vi "Autonomous Independent Vision.vi"   [LabVIEW 2016]
doc: "This VI is called when autonomous begins, and will automatically be terminated when autonomous ends. You can carry out timed or sensor driven robot movement independently without needing to return to the caller."
uses:
  Robot Global Data.vi
panel:
  # "Be sure to right-click and choose Data Operations>>Make Current Value default if you want to save the array values with the VI"
types:
  T1 = cluster{"Position":cluster{"x":sgl, "y":sgl}, "Angle":sgl, "Scale":sgl, "Score":sgl, "Bounding Box":cluster{"x":sgl, "y":sgl}[]}[]
  T2 = cluster{"Position":cluster{"x":sgl, "y":sgl}, "Angle":sgl, "Scale":sgl, "Score":sgl, "Bounding Box":cluster{"x":sgl, "y":sgl}[]}
  T3 = typedef "WPI_MotorControlDeviceRef.ctl" = cluster{"DeviceStatus":errorcluster, "Type":T4, "PWM":cluster{"PWM Channel":T5, "DeadBand":T6}, "CAN":cluster{"Device Number":u8, "SetOutput VI Ref":variant, "GetOutput VI Ref":variant, "Enable VI Ref":variant, "Disable VI Ref":variant, "Data":variant}, "Invert":bool}
  T4 = typedef "WPI_MotorControlType.ctl" = enum16{"PWM", "CAN"}
  T5 = typedef "FPGA_DIOPWMChannel.ctl" = enum8{"PWM 0", "PWM 1", "PWM 2", "PWM 3", "PWM 4", "PWM 5", "PWM 6", "PWM 7", "PWM 8", "PWM 9", "PWM MXP 0", "PWM MXP 1", "PWM MXP 2", "PWM MXP 3", "PWM MXP 4", "PWM MXP 5", "PWM MXP 6", "PWM MXP 7", "PWM MXP 8", "PWM MXP 9", "Invalid"}
  T6 = typedef "WPI_PWMDeadband.ctl" = cluster{"Name":string, "maxPositivePwm":i32, "minPositivePwm":i32, "centerPwm":i32, "maxNegativePwm":i32, "minNegativePwm":i32, "angularRange":u16}
  T7 = typedef "WPI_EncoderDevRef.ctl" = cluster{"DevStatus":errorcluster, "EncoderIndex":T8, "CounterIndex":T9, "DistancePerCount":dbl, "Decoding Type":T10}
  T8 = typedef "FPGA_EncoderIdx.ctl" = enum8{"Enc 0", "Enc 1", "Enc 2", "Enc 3", "Enc 4", "Enc 5", "Enc 6", "Enc 7", "Invalid"}
  T9 = typedef "FPGA_CounterCtrSystemIndex.ctl" = enum8{"Ctr 0", "Ctr 1", "Ctr 2", "Ctr 3", "Ctr 4", "Ctr 5", "Ctr 6", "Ctr 7", "Invalid"}
  T10 = typedef "WPI_EncoderType.ctl" = enum16{"1x", "2x", "4x"}
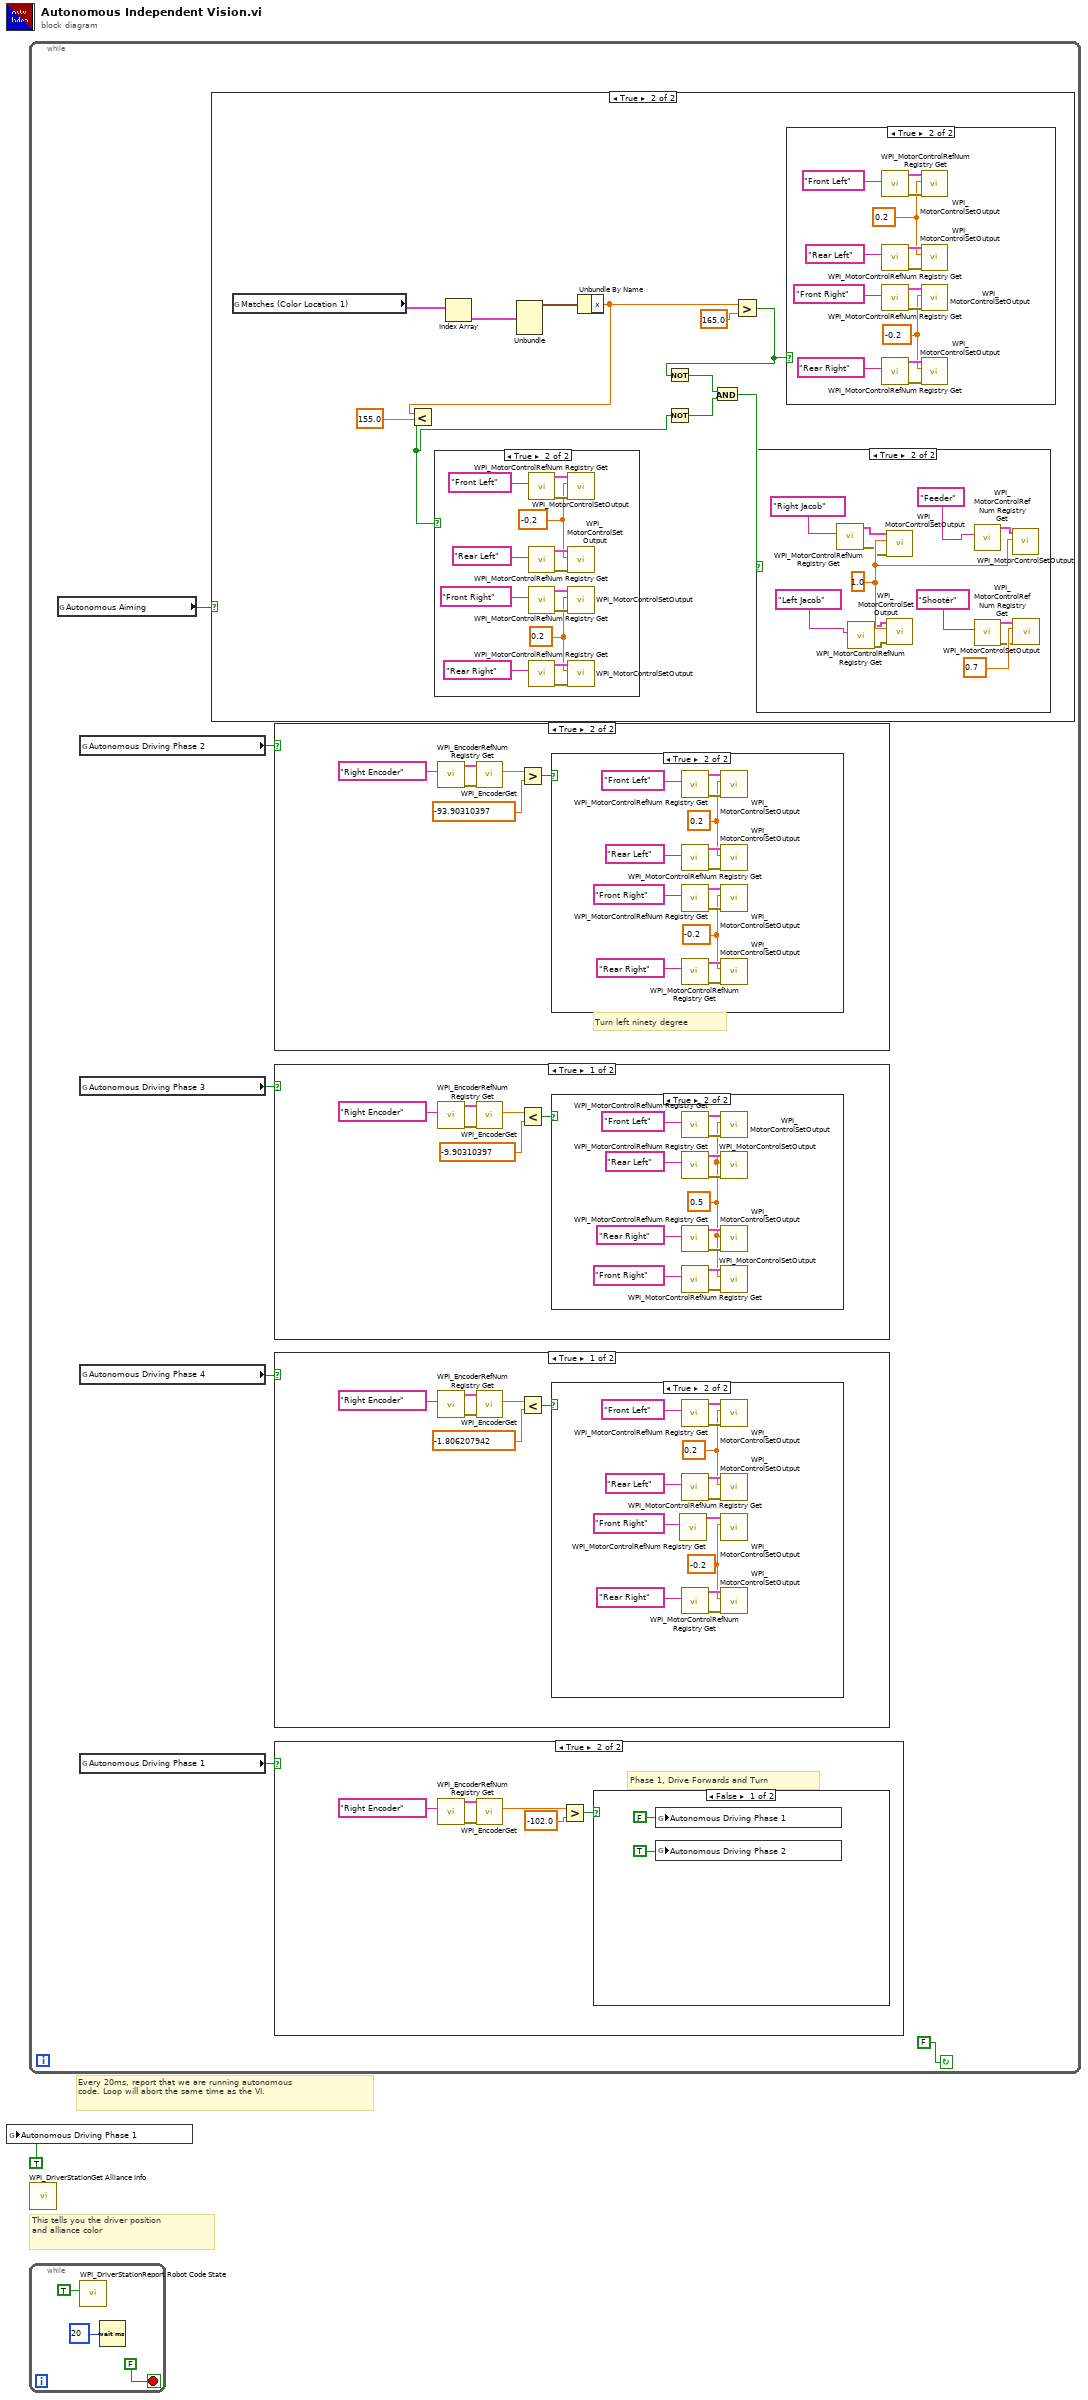
[diagram p0: block diagram]
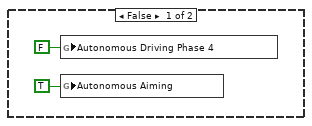
[diagram p2: hidden frame]
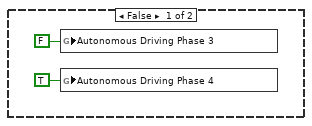
[diagram p4: hidden frame]
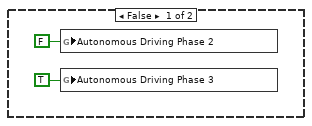
[diagram p7: hidden frame]
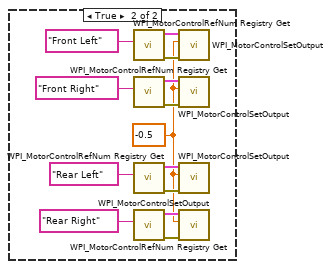
[diagram p13: hidden frame]
diagram:
  # "Every 20ms, report that we are running autonomous\ncode. Loop will abort the same time as the VI."
  # "This tells you the driver position\nand alliance color"
  n1 = global write "Robot Global Data.vi" "Autonomous Driving Phase 1"(TRUE ("Autonomous Driving")) -> ()
  n2 = while {
    stop <- FALSE continue-if-true
    n3 = global read "Robot Global Data.vi" "Autonomous Aiming"() -> (w5:bool)
    n4 = global read "Robot Global Data.vi" "Autonomous Driving Phase 2"() -> (w4:bool)
    n5 = global read "Robot Global Data.vi" "Autonomous Driving Phase 3"() -> (w3:bool)
    n6 = global read "Robot Global Data.vi" "Autonomous Driving Phase 4"() -> (w2:bool)
    n7 = global read "Robot Global Data.vi" "Autonomous Driving Phase 1"() -> (w6:bool)
    n8 = case shown="True" w5 {
      frame False {
      }
      frame True {
        n9 = global read "Robot Global Data.vi" "Matches (Color Location 1)"() -> (w82:T1)
        n10 = Index Array(array=w82) -> (element=w81:T2)  [unwired: 1 in]
        n11 = Unbundle(w81) -> ("Position"=w80:cluster{"x":sgl, "y":sgl})  [unwired: 4 out]
        n12 = Unbundle By Name(w80) -> ("x"=w78:sgl)
        n13 = Less?(x=w78, y=sgl 155.0) -> (x < y?=w75:bool)
        n14 = case shown="True" w75 {
          frame False {
          }
          frame True {
            w99 = 0.2
            w96 = -0.2
            n15 = call <vilib>:"WPI_MotorControlRefNum Registry Get.vi"("refnum name"="Front Left") -> ("error out"=w109:errorcluster, "MotorControlDevRef"=w97:T3)  [unwired: 9 in]
            n16 = call <vilib>:"WPI_MotorControlRefNum Registry Get.vi"("refnum name"="Rear Left") -> ("error out"=w105:errorcluster, "MotorControlDevRef"=w104:T3)  [unwired: 9 in]
            n17 = call <vilib>:"WPI_MotorControlRefNum Registry Get.vi"("refnum name"="Front Right") -> ("error out"=w108:errorcluster, "MotorControlDevRef"=w107:T3)  [unwired: 9 in]
            n18 = call <vilib>:"WPI_MotorControlRefNum Registry Get.vi"("refnum name"="Rear Right") -> ("error out"=w102:errorcluster, "MotorControlDevRef"=w101:T3)  [unwired: 9 in]
            n19 = call <vilib>:"WPI_MotorControlSetOutput.vi"("error in (no error)"=w109, "Output"=w96, "MotorControlDevRef"=w97) -> ()  [unwired: 6 in, 3 out]
            n20 = call <vilib>:"WPI_MotorControlSetOutput.vi"("error in (no error)"=w105, "Output"=w96, "MotorControlDevRef"=w104) -> ()  [unwired: 6 in, 3 out]
            n21 = call <vilib>:"WPI_MotorControlSetOutput.vi"("error in (no error)"=w108, "Output"=w99, "MotorControlDevRef"=w107) -> ()  [unwired: 6 in, 3 out]
            n22 = call <vilib>:"WPI_MotorControlSetOutput.vi"("error in (no error)"=w102, "Output"=w99, "MotorControlDevRef"=w101) -> ()  [unwired: 6 in, 3 out]
          }
        }
        n23 = Not(x=w75) -> (.not. x?=w73:bool)
        n24 = Greater?(x=w78, y=sgl 165.0) -> (0:w76:bool)
        n25 = Not(x=w76) -> (.not. x?=w74:bool)
        n26 = And(x=w74, y=w73) -> (x .and. y?=w72:bool)
        n27 = case shown="True" w72 {
          frame False {
          }
          frame True {
            w95 = 1.0
            n28 = call <vilib>:"WPI_MotorControlRefNum Registry Get.vi"("refnum name"="Right Jacob") -> ("error out"=w93:errorcluster, "MotorControlDevRef"=w92:T3)  [unwired: 9 in]
            n29 = call <vilib>:"WPI_MotorControlRefNum Registry Get.vi"("refnum name"="Left Jacob") -> ("error out"=w88:errorcluster, "MotorControlDevRef"=w87:T3)  [unwired: 9 in]
            n30 = call <vilib>:"WPI_MotorControlSetOutput.vi"("error in (no error)"=w93, "Output"=w95, "MotorControlDevRef"=w92) -> ()  [unwired: 6 in, 3 out]
            n31 = call <vilib>:"WPI_MotorControlSetOutput.vi"("error in (no error)"=w88, "Output"=w95, "MotorControlDevRef"=w87) -> ()  [unwired: 6 in, 3 out]
            n32 = call <vilib>:"WPI_MotorControlRefNum Registry Get.vi"("refnum name"="Feeder") -> ("MotorControlDevRef"=w89:T3)  [unwired: 9 in, 1 out]
            n33 = call <vilib>:"WPI_MotorControlRefNum Registry Get.vi"("refnum name"="Shootér") -> ("error out"=w85:errorcluster, "MotorControlDevRef"=w84:T3)  [unwired: 9 in]
            n34 = call <vilib>:"WPI_MotorControlSetOutput.vi"("Output"=w95, "MotorControlDevRef"=w89) -> ()  [unwired: 7 in, 3 out]
            n35 = call <vilib>:"WPI_MotorControlSetOutput.vi"("error in (no error)"=w85, "Output"=0.7, "MotorControlDevRef"=w84) -> ()  [unwired: 6 in, 3 out]
          }
        }
        n36 = case shown="True" w76 {
          frame False {
          }
          frame True {
            w113 = -0.2
            w110 = 0.2
            n37 = call <vilib>:"WPI_MotorControlRefNum Registry Get.vi"("refnum name"="Front Left") -> ("error out"=w123:errorcluster, "MotorControlDevRef"=w111:T3)  [unwired: 9 in]
            n38 = call <vilib>:"WPI_MotorControlRefNum Registry Get.vi"("refnum name"="Rear Left") -> ("error out"=w119:errorcluster, "MotorControlDevRef"=w118:T3)  [unwired: 9 in]
            n39 = call <vilib>:"WPI_MotorControlRefNum Registry Get.vi"("refnum name"="Front Right") -> ("error out"=w122:errorcluster, "MotorControlDevRef"=w121:T3)  [unwired: 9 in]
            n40 = call <vilib>:"WPI_MotorControlRefNum Registry Get.vi"("refnum name"="Rear Right") -> ("error out"=w116:errorcluster, "MotorControlDevRef"=w115:T3)  [unwired: 9 in]
            n41 = call <vilib>:"WPI_MotorControlSetOutput.vi"("error in (no error)"=w123, "Output"=w110, "MotorControlDevRef"=w111) -> ()  [unwired: 6 in, 3 out]
            n42 = call <vilib>:"WPI_MotorControlSetOutput.vi"("error in (no error)"=w119, "Output"=w110, "MotorControlDevRef"=w118) -> ()  [unwired: 6 in, 3 out]
            n43 = call <vilib>:"WPI_MotorControlSetOutput.vi"("error in (no error)"=w122, "Output"=w113, "MotorControlDevRef"=w121) -> ()  [unwired: 6 in, 3 out]
            n44 = call <vilib>:"WPI_MotorControlSetOutput.vi"("error in (no error)"=w116, "Output"=w113, "MotorControlDevRef"=w115) -> ()  [unwired: 6 in, 3 out]
          }
        }
      }
    }
    n45 = case shown="True" w4 {
      frame False {
      }
      frame True {
        # "Turn left ninety degree"
        n46 = call <vilib>:"WPI_EncoderRefNum Registry Get.vi"("refnum name"="Right Encoder") -> ("error out"=w54:errorcluster, "EncoderDevRef"=w53:T7)  [unwired: 9 in]
        n47 = call <vilib>:"WPI_EncoderGet.vi"("error in (no error)"=w54, "EncoderDevRef"=w53) -> ("Distance"=w52:dbl)  [unwired: 4 in, 5 out]
        n48 = Greater?(x=w52, y=-93.90310397) -> (0:w50:bool)
        n49 = case shown="True" w50 {
          frame False {
            n50 = global write "Robot Global Data.vi" "Autonomous Driving Phase 2"(FALSE ("Autonomous Driving Phase 2")) -> ()
            n51 = global write "Robot Global Data.vi" "Autonomous Driving Phase 3"(TRUE ("Autonomous Driving Phase 3")) -> ()
          }
          frame True {
            w58 = -0.2
            w59 = 0.2
            n52 = call <vilib>:"WPI_MotorControlRefNum Registry Get.vi"("refnum name"="Front Left") -> ("error out"=w71:errorcluster, "MotorControlDevRef"=w70:T3)  [unwired: 9 in]
            n53 = call <vilib>:"WPI_MotorControlRefNum Registry Get.vi"("refnum name"="Rear Left") -> ("error out"=w65:errorcluster, "MotorControlDevRef"=w64:T3)  [unwired: 9 in]
            n54 = call <vilib>:"WPI_MotorControlRefNum Registry Get.vi"("refnum name"="Front Right") -> ("error out"=w68:errorcluster, "MotorControlDevRef"=w67:T3)  [unwired: 9 in]
            n55 = call <vilib>:"WPI_MotorControlRefNum Registry Get.vi"("refnum name"="Rear Right") -> ("error out"=w62:errorcluster, "MotorControlDevRef"=w61:T3)  [unwired: 9 in]
            n56 = call <vilib>:"WPI_MotorControlSetOutput.vi"("error in (no error)"=w71, "Output"=w59, "MotorControlDevRef"=w70) -> ()  [unwired: 6 in, 3 out]
            n57 = call <vilib>:"WPI_MotorControlSetOutput.vi"("error in (no error)"=w65, "Output"=w59, "MotorControlDevRef"=w64) -> ()  [unwired: 6 in, 3 out]
            n58 = call <vilib>:"WPI_MotorControlSetOutput.vi"("error in (no error)"=w68, "Output"=w58, "MotorControlDevRef"=w67) -> ()  [unwired: 6 in, 3 out]
            n59 = call <vilib>:"WPI_MotorControlSetOutput.vi"("error in (no error)"=w62, "Output"=w58, "MotorControlDevRef"=w61) -> ()  [unwired: 6 in, 3 out]
          }
        }
      }
    }
    n60 = case shown="True" w3 {
      frame True {
        n61 = call <vilib>:"WPI_EncoderRefNum Registry Get.vi"("refnum name"="Right Encoder") -> ("error out"=w34:errorcluster, "EncoderDevRef"=w33:T7)  [unwired: 9 in]
        n62 = call <vilib>:"WPI_EncoderGet.vi"("error in (no error)"=w34, "EncoderDevRef"=w33) -> ("Distance"=w31:dbl)  [unwired: 4 in, 5 out]
        n63 = Less?(x=w31, y=-9.90310397) -> (x < y?=w29:bool)
        n64 = case shown="True" w29 {
          frame False {
            n65 = global write "Robot Global Data.vi" "Autonomous Driving Phase 3"(FALSE ("Autonomous Driving Phase 2")) -> ()
            n66 = global write "Robot Global Data.vi" "Autonomous Driving Phase 4"(TRUE ("Autonomous Driving Phase 3")) -> ()
          }
          frame True {
            w37 = 0.5
            n67 = call <vilib>:"WPI_MotorControlRefNum Registry Get.vi"("refnum name"="Front Left") -> ("error out"=w49:errorcluster, "MotorControlDevRef"=w48:T3)  [unwired: 9 in]
            n68 = call <vilib>:"WPI_MotorControlRefNum Registry Get.vi"("refnum name"="Rear Left") -> ("error out"=w43:errorcluster, "MotorControlDevRef"=w42:T3)  [unwired: 9 in]
            n69 = call <vilib>:"WPI_MotorControlRefNum Registry Get.vi"("refnum name"="Rear Right") -> ("error out"=w40:errorcluster, "MotorControlDevRef"=w39:T3)  [unwired: 9 in]
            n70 = call <vilib>:"WPI_MotorControlRefNum Registry Get.vi"("refnum name"="Front Right") -> ("error out"=w46:errorcluster, "MotorControlDevRef"=w45:T3)  [unwired: 9 in]
            n71 = call <vilib>:"WPI_MotorControlSetOutput.vi"("error in (no error)"=w49, "Output"=w37, "MotorControlDevRef"=w48) -> ()  [unwired: 6 in, 3 out]
            n72 = call <vilib>:"WPI_MotorControlSetOutput.vi"("error in (no error)"=w43, "Output"=w37, "MotorControlDevRef"=w42) -> ()  [unwired: 6 in, 3 out]
            n73 = call <vilib>:"WPI_MotorControlSetOutput.vi"("error in (no error)"=w40, "Output"=w37, "MotorControlDevRef"=w39) -> ()  [unwired: 6 in, 3 out]
            n74 = call <vilib>:"WPI_MotorControlSetOutput.vi"("error in (no error)"=w46, "Output"=w37, "MotorControlDevRef"=w45) -> ()  [unwired: 6 in, 3 out]
          }
        }
      }
      frame False {
      }
    }
    n75 = case shown="True" w2 {
      frame True {
        n76 = call <vilib>:"WPI_EncoderRefNum Registry Get.vi"("refnum name"="Right Encoder") -> ("error out"=w13:errorcluster, "EncoderDevRef"=w12:T7)  [unwired: 9 in]
        n77 = call <vilib>:"WPI_EncoderGet.vi"("error in (no error)"=w13, "EncoderDevRef"=w12) -> ("Distance"=w10:dbl)  [unwired: 4 in, 5 out]
        n78 = Less?(x=w10, y=-1.806207942) -> (x < y?=w8:bool)
        n79 = case shown="True" w8 {
          frame False {
            n80 = global write "Robot Global Data.vi" "Autonomous Driving Phase 4"(FALSE ("Autonomous Driving")) -> ()
            n81 = global write "Robot Global Data.vi" "Autonomous Aiming"(TRUE ("Autonomous Driving")) -> ()
          }
          frame True {
            w16 = -0.2
            w17 = 0.2
            n82 = call <vilib>:"WPI_MotorControlRefNum Registry Get.vi"("refnum name"="Front Right") -> ("MotorControlDevRef"=w25:T3)  [unwired: 9 in, 1 out]
            n83 = call <vilib>:"WPI_MotorControlRefNum Registry Get.vi"("refnum name"="Front Left") -> ("error out"=w28:errorcluster, "MotorControlDevRef"=w27:T3)  [unwired: 9 in]
            n84 = call <vilib>:"WPI_MotorControlRefNum Registry Get.vi"("refnum name"="Rear Left") -> ("error out"=w23:errorcluster, "MotorControlDevRef"=w22:T3)  [unwired: 9 in]
            n85 = call <vilib>:"WPI_MotorControlRefNum Registry Get.vi"("refnum name"="Rear Right") -> ("error out"=w20:errorcluster, "MotorControlDevRef"=w19:T3)  [unwired: 9 in]
            n86 = call <vilib>:"WPI_MotorControlSetOutput.vi"("error in (no error)"=w28, "Output"=w17, "MotorControlDevRef"=w27) -> ()  [unwired: 6 in, 3 out]
            n87 = call <vilib>:"WPI_MotorControlSetOutput.vi"("error in (no error)"=w23, "Output"=w17, "MotorControlDevRef"=w22) -> ()  [unwired: 6 in, 3 out]
            n88 = call <vilib>:"WPI_MotorControlSetOutput.vi"("Output"=w16, "MotorControlDevRef"=w25) -> ()  [unwired: 7 in, 3 out]
            n89 = call <vilib>:"WPI_MotorControlSetOutput.vi"("error in (no error)"=w20, "Output"=w16, "MotorControlDevRef"=w19) -> ()  [unwired: 6 in, 3 out]
          }
        }
      }
      frame False {
      }
    }
    n90 = case shown="True" w6 {
      frame False {
      }
      frame True {
        # "Phase 1, Drive Forwards and Turn"
        n91 = call <vilib>:"WPI_EncoderRefNum Registry Get.vi"("refnum name"="Right Encoder") -> ("error out"=w128:errorcluster, "EncoderDevRef"=w127:T7)  [unwired: 9 in]
        n92 = call <vilib>:"WPI_EncoderGet.vi"("error in (no error)"=w128, "EncoderDevRef"=w127) -> ("Distance"=w126:dbl)  [unwired: 4 in, 5 out]
        n93 = Greater?(x=w126, y=-102.0) -> (0:w124:bool)
        n94 = case shown="False" w124 {
          frame False {
            n95 = global write "Robot Global Data.vi" "Autonomous Driving Phase 1"(FALSE ("Autonomous Driving Phase 2")) -> ()
            n96 = global write "Robot Global Data.vi" "Autonomous Driving Phase 2"(TRUE ("Autonomous Driving Phase 2")) -> ()
          }
          frame True {
            w132 = -0.5
            n97 = call <vilib>:"WPI_MotorControlRefNum Registry Get.vi"("refnum name"="Front Left") -> ("error out"=w144:errorcluster, "MotorControlDevRef"=w143:T3)  [unwired: 9 in]
            n98 = call <vilib>:"WPI_MotorControlRefNum Registry Get.vi"("refnum name"="Front Right") -> ("error out"=w141:errorcluster, "MotorControlDevRef"=w140:T3)  [unwired: 9 in]
            n99 = call <vilib>:"WPI_MotorControlRefNum Registry Get.vi"("refnum name"="Rear Left") -> ("error out"=w138:errorcluster, "MotorControlDevRef"=w137:T3)  [unwired: 9 in]
            n100 = call <vilib>:"WPI_MotorControlRefNum Registry Get.vi"("refnum name"="Rear Right") -> ("error out"=w135:errorcluster, "MotorControlDevRef"=w134:T3)  [unwired: 9 in]
            n101 = call <vilib>:"WPI_MotorControlSetOutput.vi"("error in (no error)"=w144, "Output"=w132, "MotorControlDevRef"=w143) -> ()  [unwired: 6 in, 3 out]
            n102 = call <vilib>:"WPI_MotorControlSetOutput.vi"("error in (no error)"=w141, "Output"=w132, "MotorControlDevRef"=w140) -> ()  [unwired: 6 in, 3 out]
            n103 = call <vilib>:"WPI_MotorControlSetOutput.vi"("error in (no error)"=w138, "Output"=w132, "MotorControlDevRef"=w137) -> ()  [unwired: 6 in, 3 out]
            n104 = call <vilib>:"WPI_MotorControlSetOutput.vi"("error in (no error)"=w135, "Output"=w132, "MotorControlDevRef"=w134) -> ()  [unwired: 6 in, 3 out]
          }
        }
      }
    }
  }
  n105 = call <vilib>:"WPI_DriverStationGet Alliance Info.vi"() -> ()  [unwired: 12 out]
  n106 = while {
    stop <- FALSE stop-if-true
    n107 = call <vilib>:"WPI_DriverStationReport Robot Code State.vi"("Autonomous"=TRUE) -> ()  [unwired: 10 in, 1 out]
    n108 = Wait (ms)(milliseconds to wait=u32 20) -> ()  [unwired: 1 out]
  }
